vi "convert_mode_index_to_enum.vi"(10 "index":i32, 11 "CtlRef":refnum<vi>) -> (0 "error out":errorcluster, 1 "Usb_ports":refnum<visa-resource-name>[](array[refnum]), 2 "USB Port":refnum<visa-resource-name>, 3 "Protocol enum":T1)   [LabVIEW 2016]
uses:
  Typedef/Protocol_enum_type.ctl
panel:
  out "Strings []":string[](array[string])
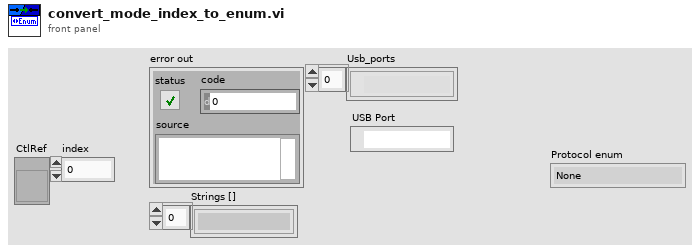
[diagram p1: front panel]
types:
  T1 = typedef "Protocol_enum_type.ctl" = enum16{"None", "MODBUS", "HART", "Fieldbus", "Profibus DP", "Profibus PA", "DeviceNET", "USB"}
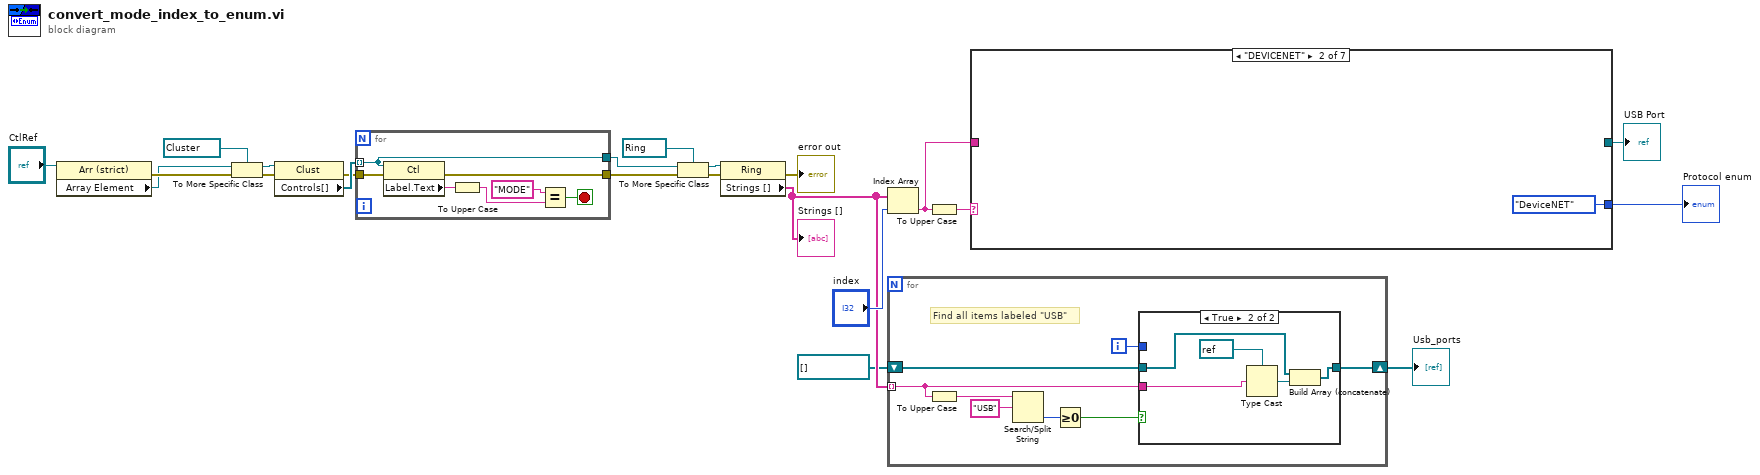
[diagram p0: block diagram]
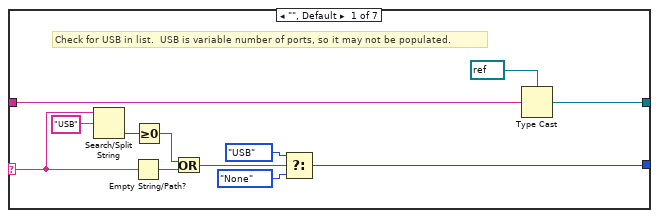
[diagram p3: hidden frame]
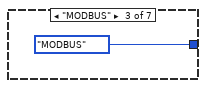
[diagram p4: hidden frame]
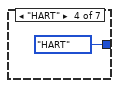
[diagram p5: hidden frame]
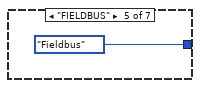
[diagram p6: hidden frame]
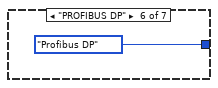
[diagram p7: hidden frame]
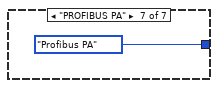
[diagram p8: hidden frame]
diagram:
  n1 = property class="Arr (strict)"(reference="CtlRef") -> (error out=w20:errorcluster, "Array Element"=w18:refnum<vi>)  [unwired: 1 in, 1 out]
  n2 = To More Specific Class(target class=refnum<vi> refnum ("Protocols"), reference=w18, error in=w20) -> (specific class reference=w16:refnum<vi>, error out=w10:errorcluster)
  n3 = property class="Clust"(reference=w16, error in=w10) -> (error out=w21:errorcluster, "Controls[]"=w22:refnum<vi>[])  [unwired: 1 out]
  n4 = for {
    tunnel: w22 -> [w25] mode=indexing
    tunnel: [w25] -> w12
    tunnel: w21 -> [w24]
    tunnel: [w23] -> w11
    stop <- w26 stop-if-true
    n5 = property class="Ctl"(reference=w25, error in=w24) -> (error out=w23:errorcluster, "Label.Text"=w29:string)  [unwired: 1 out]
    n6 = To Upper Case(1:w29) -> (0:w27:string)
    n7 = Equal?(x="MODE" ("all upper case string"), y=w27) -> (x = y?=w26:bool)
  }
  n8 = To More Specific Class(target class=refnum<vi> refnum ("Protocols"), reference=w12, error in=w11) -> (specific class reference=w14:refnum<vi>, error out=w13:errorcluster)
  n9 = property class="Ring"(reference=w14, error in=w13) -> (error out=→"error out":errorcluster, "Strings []"=w5:string[])  [unwired: 1 out]
  "Strings []" <- w5
  n10 = Index Array(array=w5, index="index") -> (element=w1:string)
  n11 = for {
    tunnel: w5 -> [w32] mode=indexing
    shift-right: [w34] -> w3
    shift-left: refnum<visa-resource-name>[] [] -> [w33]
    i -> [w30]
    # "Find all items labeled \"USB\""
    n12 = To Upper Case(1:w32) -> (0:w37:string)
    n13 = Search/Split String(string=w37, search string/char (-)="USB") -> (offset of match=w35:i32)  [unwired: 1 in, 2 out]
    n14 = Greater Or Equal To 0?(x=w35) -> (x >= 0?=w31:bool)
    n15 = case shown="True" w31 {
      tunnel: [w38 w43] -> w34
      tunnel: w33 -> [w38 w42]
      tunnel: w32 -> [_ w40]
      tunnel: w30 -> [_ _]
      frame False {
      }
      frame True {
        n16 = Type Cast(type=refnum<visa-resource-name> refnum ("MODBUS resource name"), x=w40) -> (*(type *) &x=w39:refnum<visa-resource-name>)
        n17 = Build Array (concatenate)(w42, w39) -> (w43:refnum<visa-resource-name>[])
      }
    }
  }
  "Usb_ports" <- w3
  n18 = To Upper Case(1:w1) -> (0:w7:string)
  n19 = case shown="\"DEVICENET\"" w7 {
    selector: w7 -> [w45 _ _ _ _ _ _]
    tunnel: [w52 Protocol_enum_type."DeviceNET" ("Protocols") Protocol_enum_type."MODBUS" ("t") Protocol_enum_type."HART" ("Protocols") Protocol_enum_type."Fieldbus" ("Protocols") Protocol_enum_type."Profibus DP" ("Protocols") Protocol_enum_type."Profibus PA" ("Protocols")] -> w9
    tunnel: [w50 _ _ _ _ _ _] -> w2
    tunnel: w1 -> [w49 _ _ _ _ _ _]
    frame "", Default {
      # "Check for USB in list.  USB is variable number of ports, so it may not be populated."
      n20 = Search/Split String(string=w45, search string/char (-)="USB") -> (offset of match=w54:i32)  [unwired: 1 in, 2 out]
      n21 = Empty String/Path?(string/path=w45) -> (empty?=w44:bool)
      n22 = Greater Or Equal To 0?(x=w54) -> (x >= 0?=w46:bool)
      n23 = Or(x=w46, y=w44) -> (x .or. y?=w47:bool)
      n24 = Select(t=Protocol_enum_type."USB" ("Protocols"), s=w47, f=Protocol_enum_type."None" ("Protocols")) -> (s? t:f=w52:T1)
      n25 = Type Cast(type=refnum<visa-resource-name> refnum ("MODBUS resource name"), x=w49) -> (*(type *) &x=w50:refnum<visa-resource-name>)
    }
    frame "DEVICENET" {
    }
    frame "MODBUS" {
    }
    frame "HART" {
    }
    frame "FIELDBUS" {
    }
    frame "PROFIBUS DP" {
    }
    frame "PROFIBUS PA" {
    }
  }
  "Protocol enum" <- w9
  "USB Port" <- w2
